vi "Set Notify Filter.vi"(8 "错误输入（无错误）":errorcluster, 10 "Notify Filter":i32[](array[ring]) items=["FileName"=1, "DirectoryName"=2, "Attributes"=4, "Size"=8, "LastWrite"=16, "LastAccess"=32, "CreationTime"=64, "Security"=256], 11 "FilesytemWatcher Ref In":refnum<k24>) -> (0 "错误输出":errorcluster, 3 "FilesytemWatcher Ref Out":refnum<k24>)   [LabVIEW 2012, in "FileSystem Watcher.lvlib"]
uses:
  FileSystem Watcher.lvlib
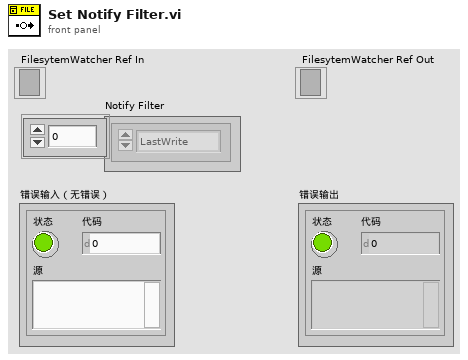
[diagram p1: front panel]
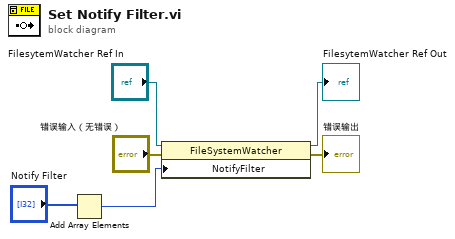
[diagram p0: block diagram]
diagram:
  n1 = Add Array Elements(numeric array="Notify Filter") -> (sum=w1:i32)
  n2 = property class="FileSystemWatcher"(reference="FilesytemWatcher Ref In", error in="错误输入（无错误）", "NotifyFilter"=w1) -> (reference out=→"FilesytemWatcher Ref Out":refnum<k24>, error out=→"错误输出":errorcluster)
